vi "Pause.vi"(8 "error in":errorcluster, 11 "4-20mA Out Settings In":T1) -> (0 "error out":errorcluster, 3 "4-20mA Out Settings Out":T1)   [LabVIEW 2018, in "Pressure Regulator Library.lvlib"]
uses:
  Pressure Regulator Library.lvlib
  Pressure Regulator Device Settings.ctl
  <vilib>/DAQmx/write.llb/DAQmx Write (Analog DBL 1Chan 1Samp).vi
  <vilib>/DAQmx/miscellaneous.llb/DAQmx Fill In Error Info.vi
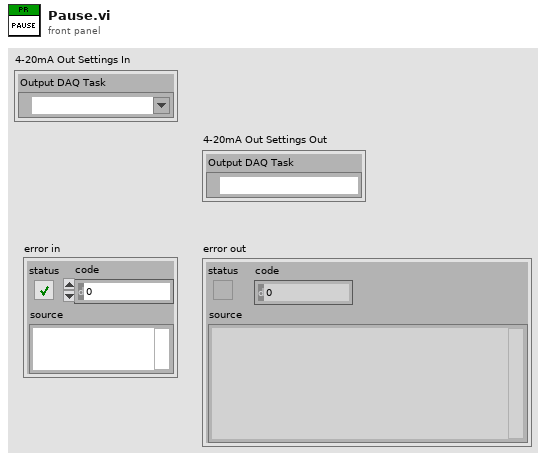
[diagram p1: front panel]
types:
  T1 = typedef "Pressure Regulator Library.lvlib/Pressure Regulator Device Settings.ctl" = cluster{"Output DAQ Task":refnum<k21>}
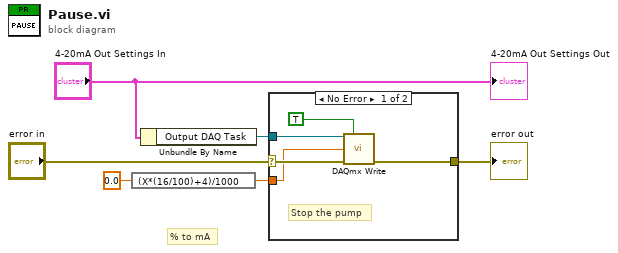
[diagram p0: block diagram]
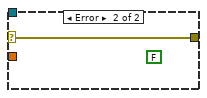
[diagram p2: hidden frame]
diagram:
  # "% to mA"
  n1 = expression code="(X*(16/100)+4)/1000"(0.0 ("speed")) -> (w6:dbl)
  n2 = Unbundle By Name("4-20mA Out Settings In") -> ("Output DAQ Task"=w5:refnum<k21>)
  n3 = case shown="No Error" "error in" {
    selector: "error in" -> [w9 w12]
    tunnel: w5 -> [w11 _]
    tunnel: w6 -> [w7 _]
    tunnel: [w8 w12] -> w2
    frame No Error {
      # "Stop the pump"
      n4 = call-poly <vilib>:"DAQmx Write.vi"("task/channels in"=w11, "auto start"=TRUE, "data"=w7, "error in"=w9) -> ("error out"=w8:errorcluster)  [unwired: 9 in, 2 out]
    }
    frame Error {
      (unwired) FALSE ("Pump On?")
    }
  }
  "error out" <- w2
  "4-20mA Out Settings Out" <- "4-20mA Out Settings In"
